vi "buildWaveform.vi"(8 "error in (no error)":errorcluster, 10 "Waveforms":T1, 11 "IWaveformFactory in":refnum<class "IWaveformFactory.lvclass">) -> (0 "error out":errorcluster, 2 "Waveform":refnum<class "IWaveform.lvclass">, 3 "IWaveformFactory out":refnum<class "IWaveformFactory.lvclass">)   [LabVIEW 2015, in "IWaveformFactory.lvclass"]
uses:
  IWaveformFactory.lvclass
  Typedefs/Waveform.ctl
  Waveforms/IWaveforms/IWaveform.lvclass
  Typedefs/FAMTTypedefs.lvlib
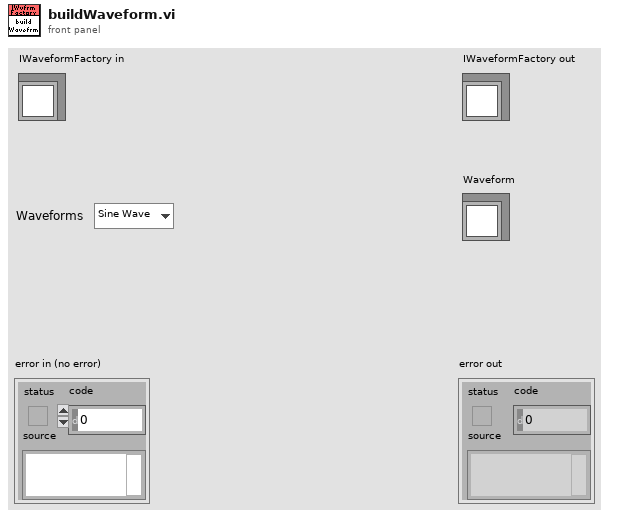
[diagram p1: front panel]
types:
  T1 = typedef "FAMTTypedefs.lvlib/Waveform.ctl" = enum16{"Sine Wave", "Triangle Wave", "Square Wave", "Sawtooth Wave", "Chirp Wave", "Gaussian Wave"}
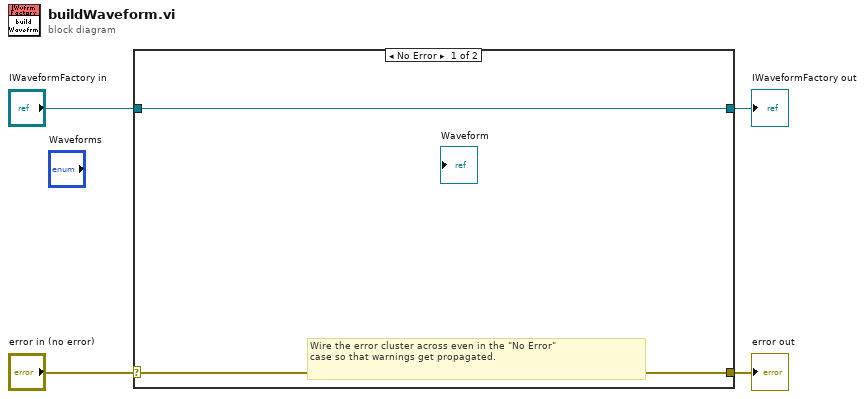
[diagram p0: block diagram]
diagram:
  n1 = case shown="No Error" "error in (no error)" {
    selector: "error in (no error)" -> [w5 w8]
    tunnel: [w5 w8] -> w3
    tunnel: [w6 w7] -> w1
    tunnel: "IWaveformFactory in" -> [w6 w7]
    frame No Error {
      # "Wire the error cluster across even in the \"No Error\"\ncase so that warnings get propagated."
    }
    frame Error {
    }
  }
  "error out" <- w3
  "IWaveformFactory out" <- w1
